vi "WSVCAP SHL Host LL RFFE Set Read_Write Parameters.vi"(0 "Transaction":T1=enum."SPI-Write/Read Data", 1 "Slave Address":u8, 5 "Wait Ticks":u32, 7 "Bytes to Write":u8, 9 "Socket Mask [U16]":u16 format="%04x", 11 "error in (no error)":errorcluster, 12 "Sub Address (Ext-Read Only)":u16 format="%04x", 13 "Bytes to Read (Ext-Read Only)":u8 format="%04x") -> (15 "error out":errorcluster)   [LabVIEW 2012]
uses:
  Type Defs/WSVCAP SHL Transaction Enum.ctl
  Type Defs/WSVCAP SHL Top Level Control Operation Enum.ctl
  Type Defs/WSVCAP SHL State.ctl
  Type Defs/WSVCAP SHL Top Level Control Enum.ctl
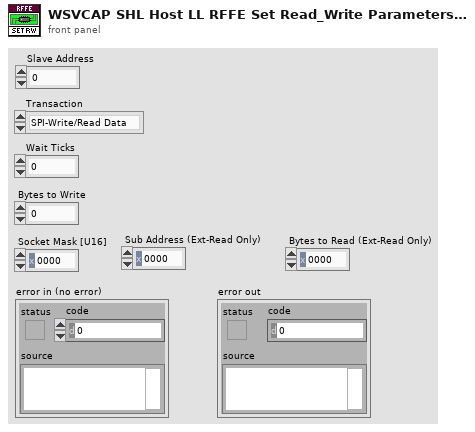
[diagram p1: front panel]
types:
  T1 = typedef "WSVCAP SHL Transaction Enum.ctl" = enum16{"I2C-Read Data", "I2C-Write Data", "SPI-Write/Read Data", "RFFE-Ext Write", "RFFE-Ext Read"}
  T2 = typedef "WSVCAP SHL Top Level Control Operation Enum.ctl" = enum16{"Initialize", "Set Control", "Read Control", "Close"}
  T3 = typedef "WSVCAP SHL State.ctl" = enum8{"Idle", "Transfer Data"}
  T4 = typedef "WSVCAP SHL Top Level Control Enum.ctl" = enum16{"Start", "Cmd", "Transaction", "Wait Ticks", "Socket Mask", "Slave Address", "Sub Address", "Bytes to Write", "Bytes to Read", "Write Data", "Write Flag", "Read Data", "Read Flag", "Ack Read", "Read Status Flag", "Ack Read Status", "Status", "Cycle Count", "Stop Cycle", "Exit"}
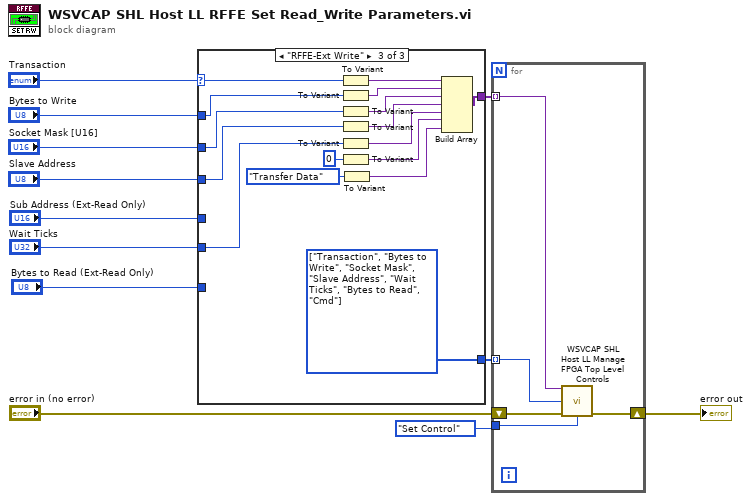
[diagram p0: block diagram]
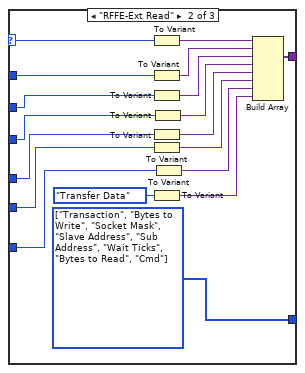
[diagram p3: hidden frame]
diagram:
  n1 = case shown="\"RFFE-Ext Write\"" "Transaction" {
    selector: "Transaction" -> [_ w19 w35]
    tunnel: [_ w27 w43] -> w11
    tunnel: [_ w25 w41] -> w8
    tunnel: "Socket Mask [U16]" -> [_ w24 w40]
    tunnel: "Bytes to Write" -> [_ w22 w38]
    tunnel: "Wait Ticks" -> [_ w21 w37]
    tunnel: "Sub Address (Ext-Read Only)" -> [_ w18 _]
    tunnel: "Slave Address" -> [_ w16 w34]
    tunnel: "Bytes to Read (Ext-Read Only)" -> [_ w14 _]
    frame Default {
    }
    frame "RFFE-Ext Read" {
      w25 = T4[] [enum."Transaction", enum."Bytes to Write", enum."Socket Mask", enum."Slave Address", enum."Sub Address", enum."Wait Ticks", enum."Bytes to Read", enum."Cmd"] items=["Start", "Cmd", "Transaction", "Wait Ticks", "Socket Mask", "Slave Address", "Sub Address", "Bytes to Write", "Bytes to Read", "Write Data", "Write Flag", "Read Data", "Read Flag", "Ack Read", "Read Status Flag", "Ack Read Status", "Status", "Cycle Count", "Stop Cycle", "Exit"]
      n2 = To Variant(anything=w19) -> (Variant=w29:variant)
      n3 = To Variant(anything=w22) -> (Variant=w28:variant)
      n4 = To Variant(anything=w24) -> (Variant=w23:variant)
      n5 = To Variant(anything=w18) -> (Variant=w17:variant)
      n6 = To Variant(anything=w21) -> (Variant=w20:variant)
      n7 = To Variant(anything=WSVCAP_SHL_State."Transfer Data" ("SPI_Cmd")) -> (Variant=w26:variant)
      n8 = To Variant(anything=w16) -> (Variant=w15:variant)
      n9 = To Variant(anything=w14) -> (Variant=w13:variant)
      n10 = Build Array(w29, w28, w23, w15, w17, w20, w13, w26) -> (w27:variant[])
    }
    frame "RFFE-Ext Write" {
      w41 = T4[] [enum."Transaction", enum."Bytes to Write", enum."Socket Mask", enum."Slave Address", enum."Wait Ticks", enum."Bytes to Read", enum."Cmd"] items=["Start", "Cmd", "Transaction", "Wait Ticks", "Socket Mask", "Slave Address", "Sub Address", "Bytes to Write", "Bytes to Read", "Write Data", "Write Flag", "Read Data", "Read Flag", "Ack Read", "Read Status Flag", "Ack Read Status", "Status", "Cycle Count", "Stop Cycle", "Exit"]
      n11 = To Variant(anything=w35) -> (Variant=w45:variant)
      n12 = To Variant(anything=w38) -> (Variant=w44:variant)
      n13 = To Variant(anything=w40) -> (Variant=w39:variant)
      n14 = To Variant(anything=w34) -> (Variant=w33:variant)
      n15 = To Variant(anything=w37) -> (Variant=w36:variant)
      n16 = To Variant(anything=u8 0 ("Bytes to Read (Ext-Read Only)")) -> (Variant=w32:variant)
      n17 = To Variant(anything=WSVCAP_SHL_State."Transfer Data" ("SPI_Cmd")) -> (Variant=w42:variant)
      n18 = Build Array(w45, w44, w39, w33, w36, w32, w42) -> (w43:variant[])
    }
  }
  n19 = for {
    tunnel: WSVCAP_SHL_Top_Level_Control_Operation_Enum."Set Control" ("Operation") -> [w51]
    tunnel: w11 -> [w50] mode=indexing
    tunnel: w8 -> [w49] mode=indexing
    shift-right: [w47] -> w9
    shift-left: "error in (no error)" -> [w48]
    n20 = call "WSVCAP SHL Host LL Manage FPGA Top Level Controls.vi"("Value In"=w50, "FPGA Top Level Control"=w49, "error in (no error)"=w48, "Operation"=w51) -> ("error out"=w47:errorcluster)  [unwired: 10 in, 1 out]
  }
  "error out" <- w9
